vi "Temperature Conversion.vi"(9 "Calibration Coefficients":dbl[](array[numeric]), 10 "Wavelength Offset (0 nm)":dbl format="%#_10g", 11 "Current Wavelength (0 nm)":dbl format="%#_10g") -> (2 "Temperature (°C)":dbl)   [LabVIEW 2015, in "Micron Optics sm130.lvlib"]
doc: "Converts the wavelength shift to absolute temperature in celcius.\n\n<b>Note:</b>\n1.) This conversion VI is compatible with Micron Optics sensor model os4200 and os4300.\n2.) Refer to the Sensor Information Sheet provided with each sensor for the constants."
uses:
  Micron Optics sm130.lvlib
panel:
  # "This conversion VI is compatible with Micron Optics sensor model os4200 and os4300."
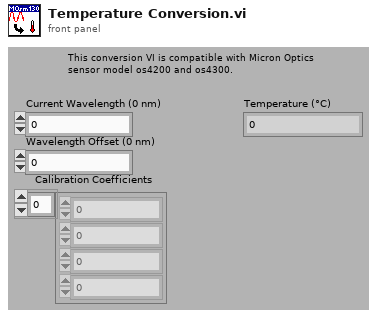
[diagram p1: front panel]
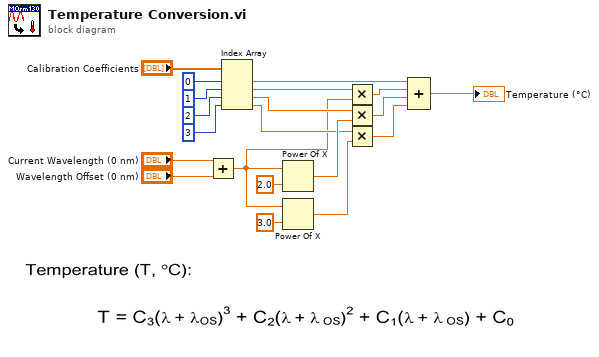
[diagram p0: block diagram]
diagram:
  n1 = Add(x="Current Wavelength (0 nm)", y="Wavelength Offset (0 nm)") -> (x+y=w2:dbl)
  n2 = Index Array(array="Calibration Coefficients", index #1=0 ("index"), index #2=1 ("index"), index #3=2 ("index"), index #4=3 ("index")) -> (element #1=w11:dbl, element #2=w9:dbl, element #3=w8:dbl, element #4=w6:dbl)
  n3 = Power Of X(1:2.0 ("x"), 2:w2) -> (0:w7:dbl)
  n4 = Power Of X(1:3.0 ("x"), 2:w2) -> (0:w5:dbl)
  n5 = Multiply(x=w9, y=w2) -> (x*y=w10:dbl)
  n6 = Multiply(x=w8, y=w7) -> (x*y=w4:dbl)
  n7 = Multiply(x=w6, y=w5) -> (x*y=w3:dbl)
  n8 = Compound Arithmetic op=ADD(w11, w10, w4, w3) -> (→"Temperature (°C)":dbl)
